vi "PicoScopeospaGetTriggerInfo.vi"(0 "handle in":i16, 5 "Segment Range":T1={"fromSegmentIndex"=0, "toSegmentIndex"=9} {"toSegmentIndex" format="%.4p"; "fromSegmentIndex" format="%.4p"}, 9 "Sample Rate":dbl, 11 "error in":errorcluster) -> (4 "handle out":i16, 6 "Trigger Info":T2(array[cluster]), 10 "Trigger Offsets":cluster{"Samples":u64, "Time (seconds)":dbl}[](array[cluster]) {"Time (seconds)" format="%#_5p"}, 15 "error out":errorcluster)   [LabVIEW 2010]
doc: "This VI gets a set of blocks captured using rapid block mode. It outputs two-dimensional arrays for each channel that contain data from all the requested captures."
uses:
  psospa.dll
  shared/Segment Range.ctl
panel:
  out "Number of Captures":u64=1
  out "fromSegmentIndex":u64
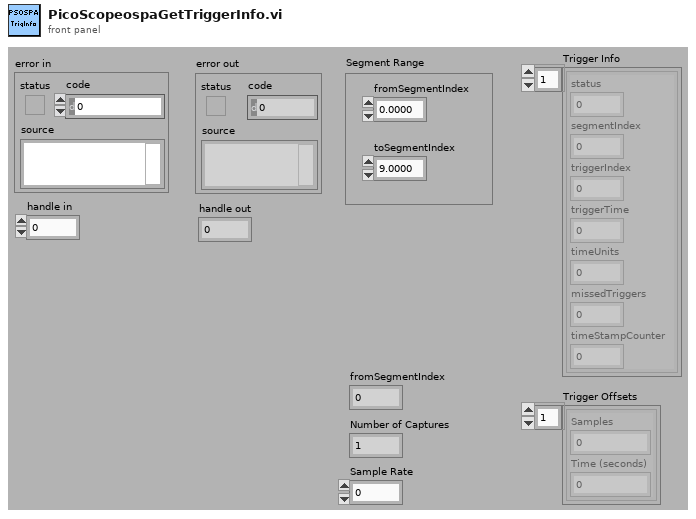
[diagram p1: front panel]
types:
  T1 = typedef "Segment Range.ctl" = cluster{"fromSegmentIndex":u64, "toSegmentIndex":u64}
  T2 = cluster{"status":u32, "segmentIndex":u64, "triggerIndex":u64, "triggerTime":dbl, "timeUnits":u32, "missedTriggers":u64, "timeStampCounter":u64}[]
  T3 = cluster{"status":u32, "segmentIndex":u64, "triggerIndex":u64, "triggerTime":dbl, "timeUnits":u32, "missedTriggers":u64, "timeStampCounter":u64}
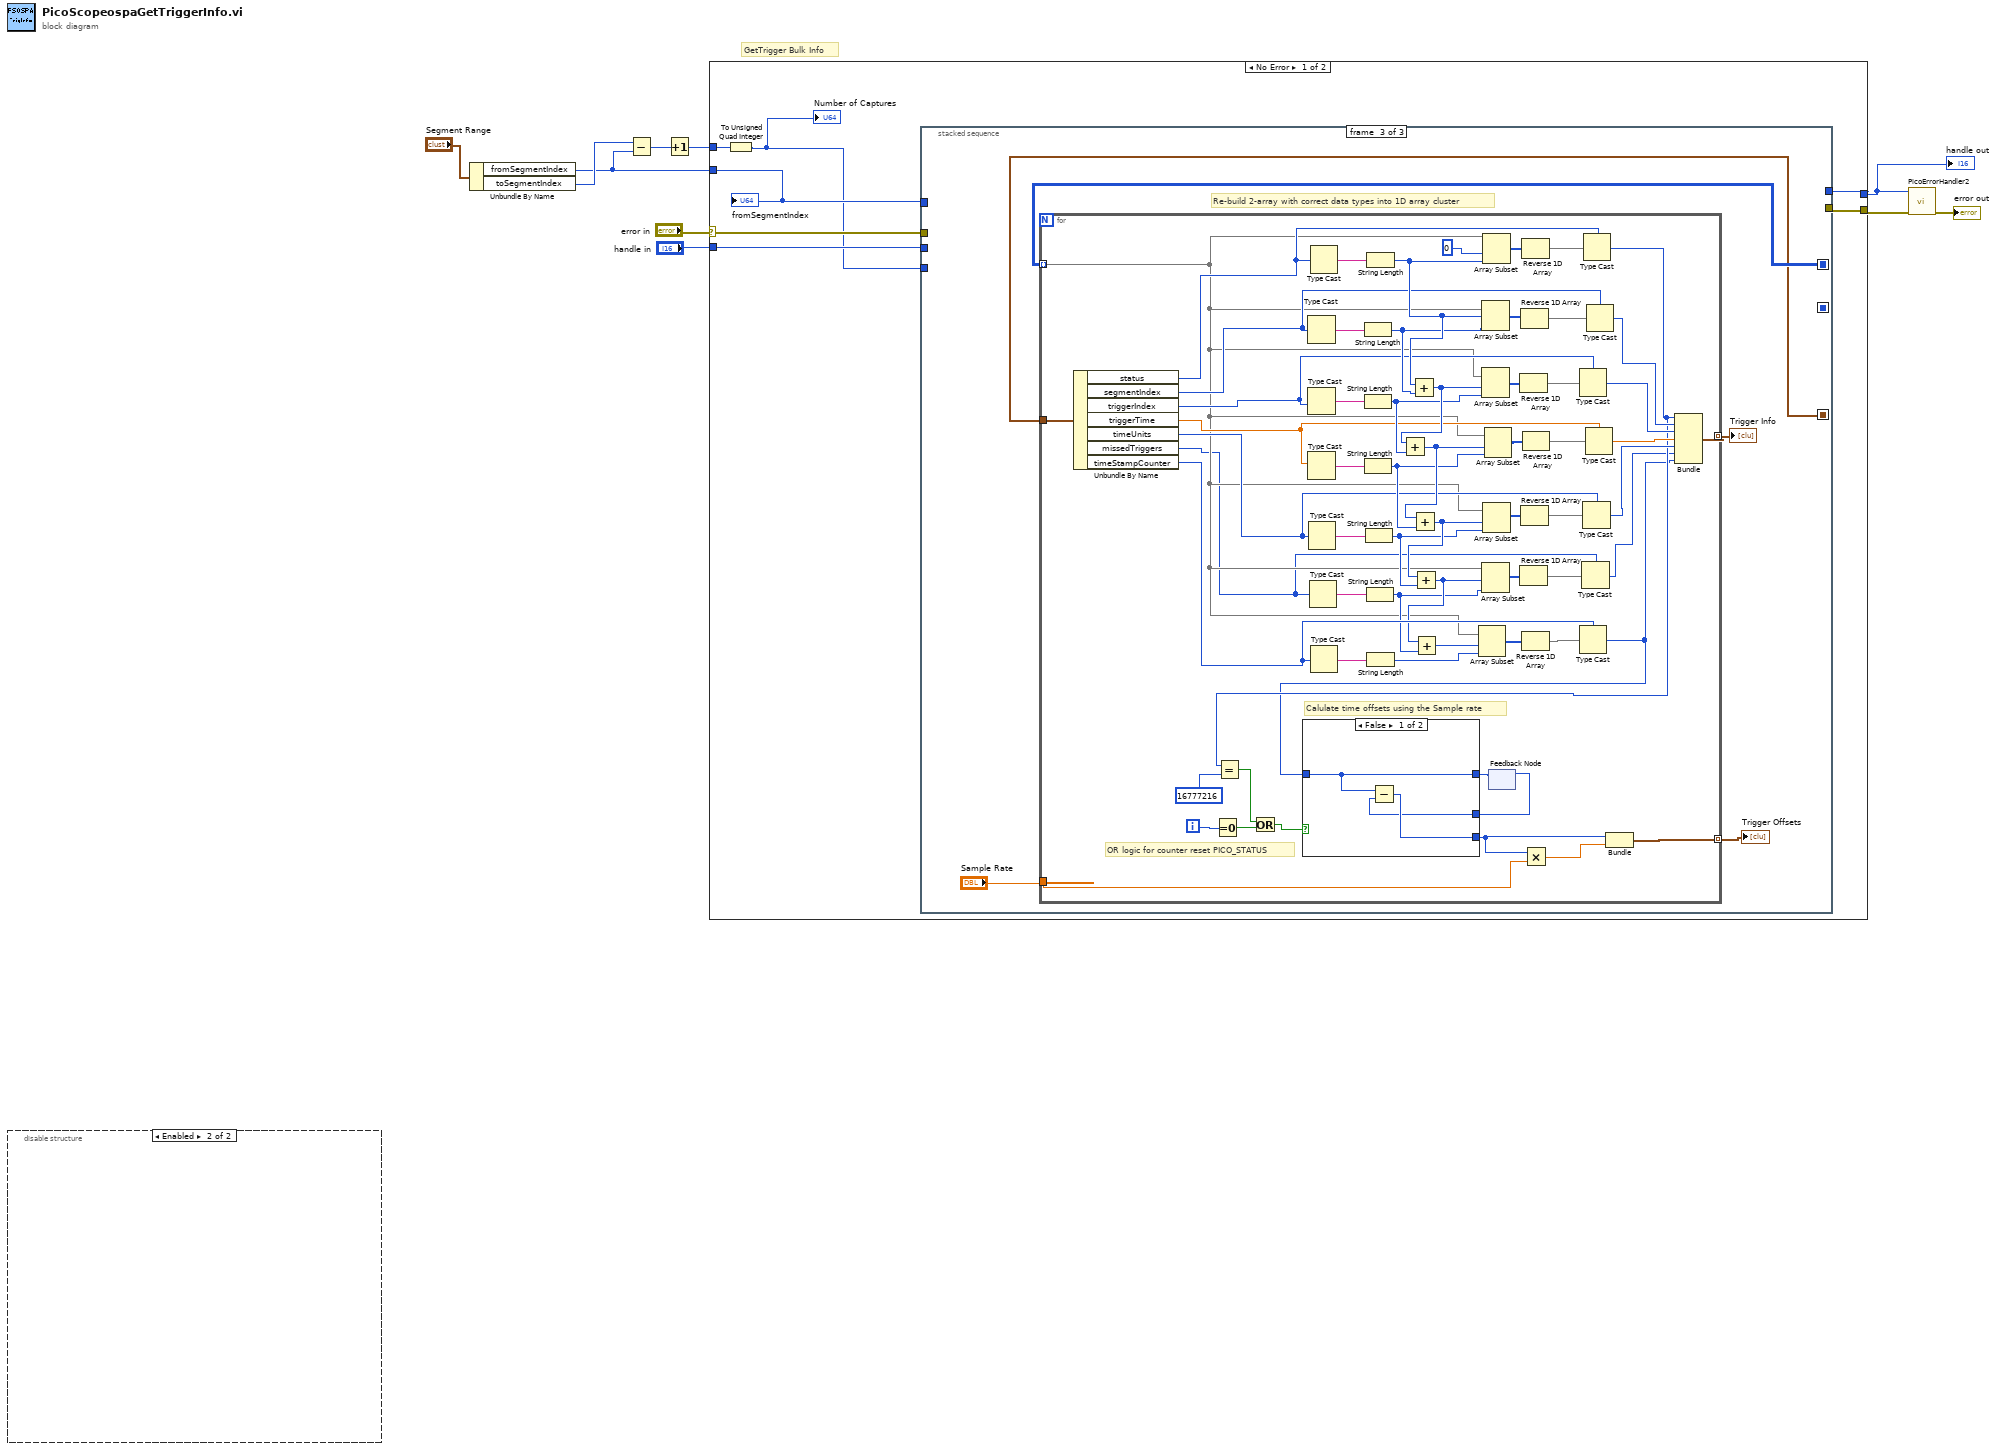
[diagram p0: block diagram]
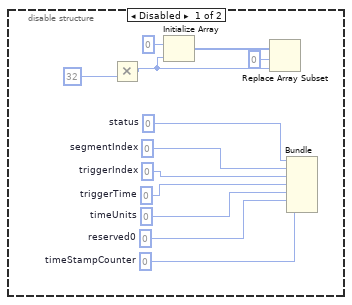
[diagram p2: hidden frame]
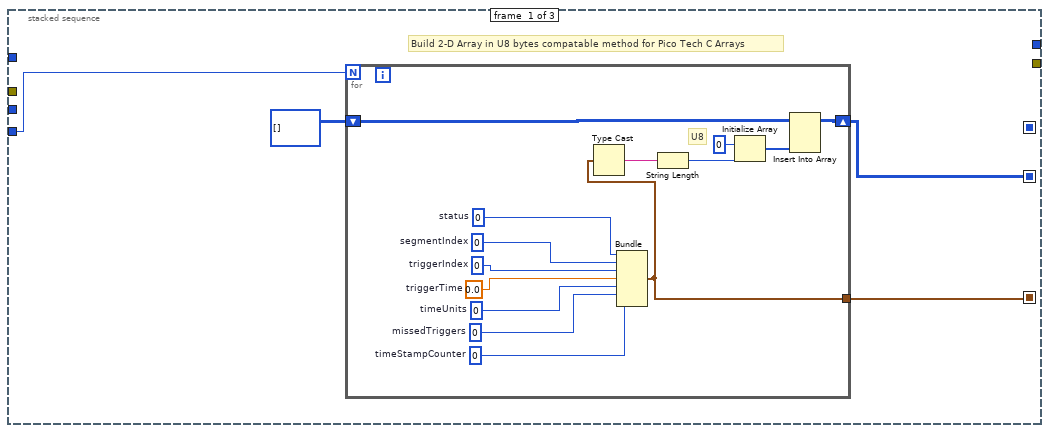
[diagram p3: hidden frame]
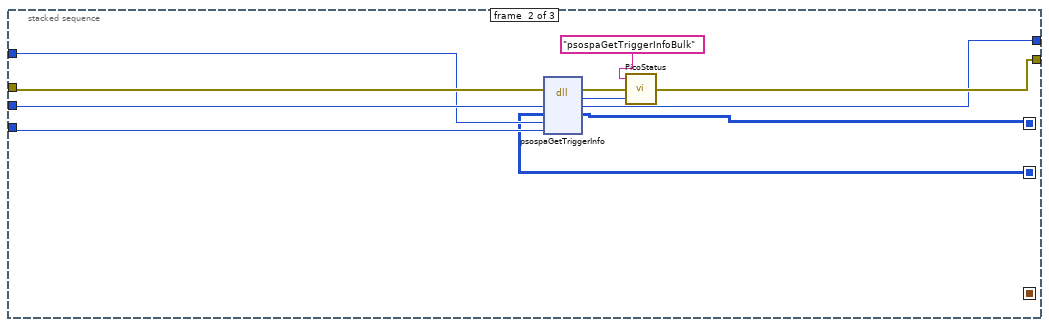
[diagram p4: hidden frame]
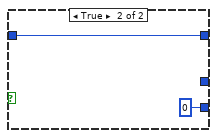
[diagram p5: hidden frame]
diagram:
  # "GetTrigger Bulk Info"
  n1 = disable-structure shown="Enabled" {
    frame Disabled {
      w18 = u64 0  # timeStampCounter
      w16 = i16 0  # reserved0
      w17 = i16 0  # timeUnits
      w19 = i64 0  # triggerTime
      w20 = u32 0  # triggerIndex
      w21 = u32 0  # segmentIndex
      w22 = u32 0  # status
      n2 = Multiply(y=u32 32) -> (x*y=w14:u32)  [unwired: 1 in]
      n3 = Initialize Array(u8 0 ("element"), w14) -> (w15:u8[])
      n4 = Replace Array Subset(array=w15, new element=w14, index=0) -> ()  [unwired: 1 out]
      n5 = Bundle("status"=w22, "segmentIndex"=w21, "triggerIndex"=w20, "triggerTime"=w19, "timeUnits"=w17, "reserved0"=w16, "timeStampCounter"=w18) -> ()  [unwired: 1 in, 1 out]
    }
    frame Enabled {
    }
  }
  n6 = Unbundle By Name("Segment Range") -> ("fromSegmentIndex"=w4:u64, "toSegmentIndex"=w5:u64)
  n7 = Subtract(x=w5, y=w4) -> (x-y=w3:u64)
  n8 = Increment(x=w3) -> (x+1=w2:u64)
  n9 = case shown="No Error" "error in" {
    selector: "error in" -> [w29 w133]
    tunnel: [w27 w133] -> w7
    tunnel: "handle in" -> [w28 w132]
    tunnel: [w26 w132] -> w8
    tunnel: w2 -> [w25 _]
    tunnel: w4 -> [w24 _]
    frame No Error {
      n10 = To Unsigned Quad Integer(1:w25) -> (0:w23:u64)
      "Number of Captures" <- w23
      n11 = stacked-sequence {
        seq-local: [w32 _ _] -> [_ w51 _]
        seq-local: [w31 _ _] -> [_ w49 _]
        seq-local: [_ w50 _] -> [_ _ w64]
        seq-local: [_ w49 _] -> [_ _ w61]
        tunnel: w29 -> [_ w56 _]
        tunnel: w28 -> [_ w54 _]
        tunnel: w24 -> [_ w53 _]
        tunnel: w23 -> [w30 w52 _]
        tunnel: [_ w55 _] -> w27
        tunnel: [_ w48 _] -> w26
        frame #0 {
          # "Build 2-D Array in U8 bytes compatable method for Pico Tech C Arrays"
          n12 = for {
            N: w30 -> [_]
            shift-right: [w35] -> w32
            shift-left: u8[][] [] -> [w36]
            tunnel: [w34] -> w31
            w43 = u64 0  # timeStampCounter
            w41 = u64 0  # missedTriggers
            w42 = u32 0  # timeUnits
            w44 = 0.0  # triggerTime
            w45 = u64 0  # triggerIndex
            w46 = u64 0  # segmentIndex
            w47 = u32 0  # status
            # "U8"
            n13 = Bundle("status"=w47, "segmentIndex"=w46, "triggerIndex"=w45, "triggerTime"=w44, "timeUnits"=w42, "missedTriggers"=w41, "timeStampCounter"=w43) -> (w34:T3)  [unwired: 1 in]
            n14 = Type Cast(x=w34) -> (*(type *) &x=w40:string)  [unwired: 1 in]
            n15 = String Length(string=w40) -> (length=w38:i32)
            n16 = Initialize Array(u8 0 ("element"), w38) -> (w37:u8[])
            n17 = Insert Into Array(array=w36, new element=w37) -> (w35:u8[][])  [unwired: 2 in]
          }
        }
        frame #1 {
          n18 = dll-call lib="psospa.dll" fn="psospaGetTriggerInfo" ("ps3000.dll:_ps3000_open_unit@0")(error in=w56, "handle"=w54, "triggerInfo"=w51, "firstSegmentIndex"=w53, "segmentCount"=w52) -> (error out=w59:errorcluster, "PICO_STATUS"=w58:u32, "handle"=w48:i16, "triggerInfo"=w50:u8[][])  [unwired: 4 in, 1 out]
          n19 = call "PicoStatus.vi"("PICO STATUS"=w58, "error in"=w59, "source"="psospaGetTriggerInfoBulk") -> ("error out"=w55:errorcluster)
        }
        frame #2 {
          # "Re-build 2-array with correct data types into 1D array cluster"
          n20 = for {
            tunnel: w64 -> [w67] mode=indexing
            tunnel: [w123] -> w60 mode=indexing
            tunnel: [w107] -> w63 mode=indexing
            tunnel: "Sample Rate" -> [w106]
            tunnel: w61 -> [w79]
            i -> [w110]
            # "Calulate time offsets using the Sample rate"
            # "OR logic for counter reset PICO_STATUS"
            n21 = Unbundle By Name(w79) -> ("status"=w78:u32, "segmentIndex"=w77:u64, "triggerIndex"=w73:u64, "triggerTime"=w74:dbl, "timeUnits"=w75:u32, "missedTriggers"=w66:u64, "timeStampCounter"=w76:u64)
            n22 = Equal To 0?(x=w110) -> (x = 0?=w84:bool)
            n23 = Type Cast(x=w77) -> (*(type *) &x=w102:string)  [unwired: 1 in]
            n24 = Type Cast(x=w73) -> (*(type *) &x=w101:string)  [unwired: 1 in]
            n25 = Type Cast(x=w74) -> (*(type *) &x=w100:string)  [unwired: 1 in]
            n26 = Type Cast(x=w75) -> (*(type *) &x=w99:string)  [unwired: 1 in]
            n27 = Type Cast(x=w66) -> (*(type *) &x=w98:string)  [unwired: 1 in]
            n28 = Type Cast(x=w78) -> (*(type *) &x=w103:string)  [unwired: 1 in]
            n29 = Type Cast(x=w76) -> (*(type *) &x=w93:string)  [unwired: 1 in]
            n30 = String Length(string=w102) -> (length=w89:i32)
            n31 = String Length(string=w101) -> (length=w87:i32)
            n32 = String Length(string=w100) -> (length=w86:i32)
            n33 = String Length(string=w99) -> (length=w85:i32)
            n34 = String Length(string=w98) -> (length=w70:i32)
            n35 = String Length(string=w103) -> (length=w94:i32)
            n36 = String Length(string=w93) -> (length=w91:i32)
            n37 = Add(x=w94, y=w89) -> (x+y=w88:i32)
            n38 = Add(x=w88, y=w87) -> (x+y=w97:i32)
            n39 = Add(x=w97, y=w86) -> (x+y=w96:i32)
            n40 = Add(x=w96, y=w85) -> (x+y=w71:i32)
            n41 = Add(x=w71, y=w70) -> (x+y=w92:i32)
            n42 = Array Subset(array=w67, index=w92, length=w91) -> (w90:u8[])
            n43 = Array Subset(array=w67, index=w94, length=w89) -> (w122:u8[])
            n44 = Array Subset(array=w67, index=w88, length=w87) -> (w117:u8[])
            n45 = Array Subset(array=w67, index=w71, length=w70) -> (w68:u8[])
            n46 = Array Subset(array=w67, index=0, length=w94) -> (w120:u8[])
            n47 = Array Subset(array=w67, index=w96, length=w85) -> (w114:u8[])
            n48 = Array Subset(array=w67, index=w97, length=w86) -> (w116:u8[])
            n49 = feedback #1() -> (w108:u64)  [unwired: 1 in]
            n50 = Reverse 1D Array(array=w117) -> (reversed array=w118:u8[])
            n51 = Reverse 1D Array(array=w68) -> (reversed array=w69:u8[])
            n52 = Reverse 1D Array(array=w122) -> (reversed array=w121:u8[])
            n53 = Reverse 1D Array(array=w114) -> (reversed array=w113:u8[])
            n54 = Reverse 1D Array(array=w120) -> (reversed array=w119:u8[])
            n55 = Reverse 1D Array(array=w90) -> (reversed array=w112:u8[])
            n56 = Reverse 1D Array(array=w116) -> (reversed array=w115:u8[])
            n57 = Type Cast(type=w73, x=w118) -> (*(type *) &x=w126:u64)
            n58 = Type Cast(type=w76, x=w112) -> (*(type *) &x=w72:u64)
            n59 = Type Cast(type=w66, x=w69) -> (*(type *) &x=w65:u64)
            n60 = Type Cast(type=w75, x=w113) -> (*(type *) &x=w124:u32)
            n61 = Type Cast(type=w78, x=w119) -> (*(type *) &x=w80:u32)
            n62 = Equal?(x=w80, y=u32 16777216 ("status")) -> (x = y?=w82:bool)
            n63 = Or(x=w82, y=w84) -> (x .or. y?=w83:bool)
            n64 = case shown="False" w83 {
              tunnel: w72 -> [w128 w131]
              tunnel: [w128 w131] -> w109
              tunnel: w108 -> [w127 _]
              tunnel: [w129 u64 0] -> w105
              frame False {
                n65 = Subtract(x=w128, y=w127) -> (x-y=w129:u64)
              }
              frame True {
              }
            }
            n66 = feedback-in #1(w109) -> ()
            n67 = Multiply(x=w105, y=w106) -> (x*y=w104:dbl)
            n68 = Type Cast(type=w74, x=w115) -> (*(type *) &x=w125:dbl)
            n69 = Type Cast(type=w77, x=w121) -> (*(type *) &x=w111:u64)
            n70 = Bundle(w105, w104) -> (w107:cluster{u64, dbl})  [unwired: 1 in]
            n71 = Bundle("status"=w80, "segmentIndex"=w111, "triggerIndex"=w126, "triggerTime"=w125, "timeUnits"=w124, "missedTriggers"=w65, "timeStampCounter"=w72) -> (w123:T3)  [unwired: 1 in]
          }
          "Trigger Offsets" <- w63
          "Trigger Info" <- w60
        }
      }
      "fromSegmentIndex" <- w24
    }
    frame Error {
    }
  }
  "handle out" <- w8
  n72 = call "PicoErrorHandler2.vi"("error in (no error)"=w7, "handle In"=w8) -> ("error out"=→"error out":errorcluster)  [unwired: 9 in]
